vi "PXI_Host_Cluster_Read_NewMethod_Benchmark.vi"() -> ()   [LabVIEW 2018]
uses:
  cRIO RT/TypeDefs/Simple cluster.ctl
  7e8a9f0d-2b7c-4c85-8fb4-747e2fea878c.vi
  cRIO RT/FPGA Bitfile Register Operations/Scalar IO Operations/SubVIs/Convert Cluster BLOB to Bool Array.vi
  cRIO RT/FPGA Bitfile Register Operations/Scalar IO Operations/SubVIs/Parse Cluster Configuration.vi
  cRIO RT/FPGA Bitfile Register Operations/Scalar IO Operations/Read Methods/Read Data Register/Instances/Read U8 Array.vi
  7e8a9f0d-2b7c-4c85-8fb4-747e2fea878c.vi/98fed1db-7537-4d17-af2e-83a63eeec4d6.vi
  cRIO RT/FPGA Bitfile Register Operations/Scalar IO Operations/SubVIs/Check Cluster Configuration Store.vi
  cRIO RT/FPGA Bitfile Register Operations/Scalar IO Operations/Utilities/Find Register Offset.vi
  cRIO RT/FPGA Bitfile Register Operations/Scalar IO Operations/SubVIs/FXP Raw to DBL.vi
  cRIO RT/FPGA Bitfile Register Operations/Scalar IO Operations/SubVIs/Check Register Data Store.vi
  <userlib>/_OpenG.lib/lvdata/lvdata.llb/Variant to Header Info__ogtk.vi
  <userlib>/_OpenG.lib/lvdata/lvdata.llb/Split Cluster TD__ogtk.vi
  <userlib>/_OpenG.lib/lvdata/lvdata.llb/Cluster to Array of VData__ogtk.vi
  <vilib>/Utility/Data Type/Get Type Information.vi
  <userlib>/_OpenG.lib/lvdata/lvdata.llb/Get Strings from Enum__ogtk.vi
  cRIO RT/FPGA Bitfile Register Operations/Scalar IO Operations/Error Handling/Error 6004.vi
  <vilib>/Utility/Data Type/Get Fixed-Point Information.vi
  cRIO RT/FPGA Bitfile Register Operations/Scalar IO Operations/Error Handling/Error 6001.vi
  cRIO RT/FPGA Bitfile Register Operations/Scalar IO Operations/Error Handling/Error 6000.vi
  cRIO RT/FPGA Bitfile Register Operations/Scalar IO Operations/Error Handling/Error 6002.vi
  cRIO RT/FPGA Bitfile Register Operations/Scalar IO Operations/Error Handling/Error 6003.vi
  <vilib>/FPGAPlugInAG/Dynamic/niLvFpga_Close_Dynamic.vi
  <vilib>/rvi/interface/nirviCloseFPGA/nirviCloseFPGA.xnode
  cRIO RT/FPGA Bitfile Register Operations/Scalar IO Operations/FPGA Register IO.lvlib
panel:
  out "error out":errorcluster
  out "Value out":T1
  out "Execution time (s)":dbl
  # "Recorded time"
  # "3.37551E-5"
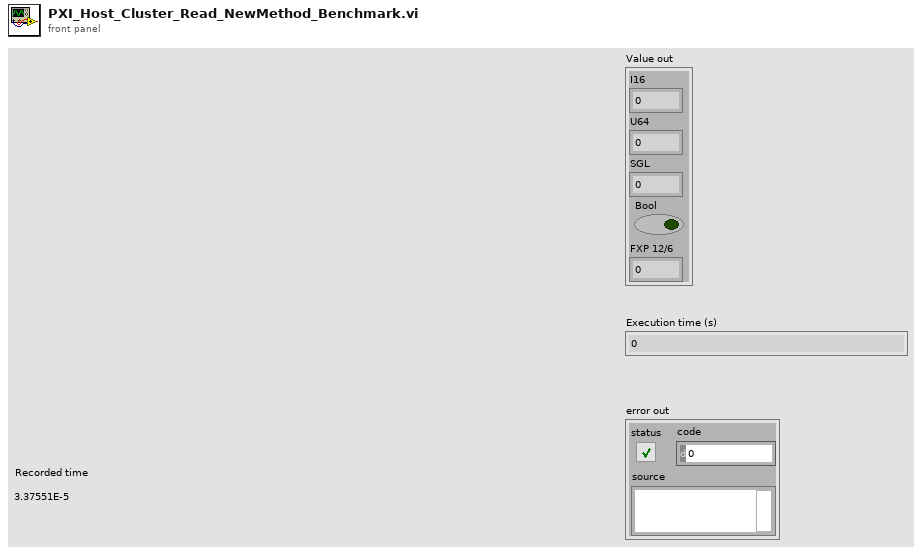
[diagram p1: front panel]
types:
  T1 = typedef "Simple cluster.ctl" = cluster{"I16":i16, "U64":u64, "SGL":sgl, "Bool":bool, "FXP 12/6":fxp<+/-,12,6>}
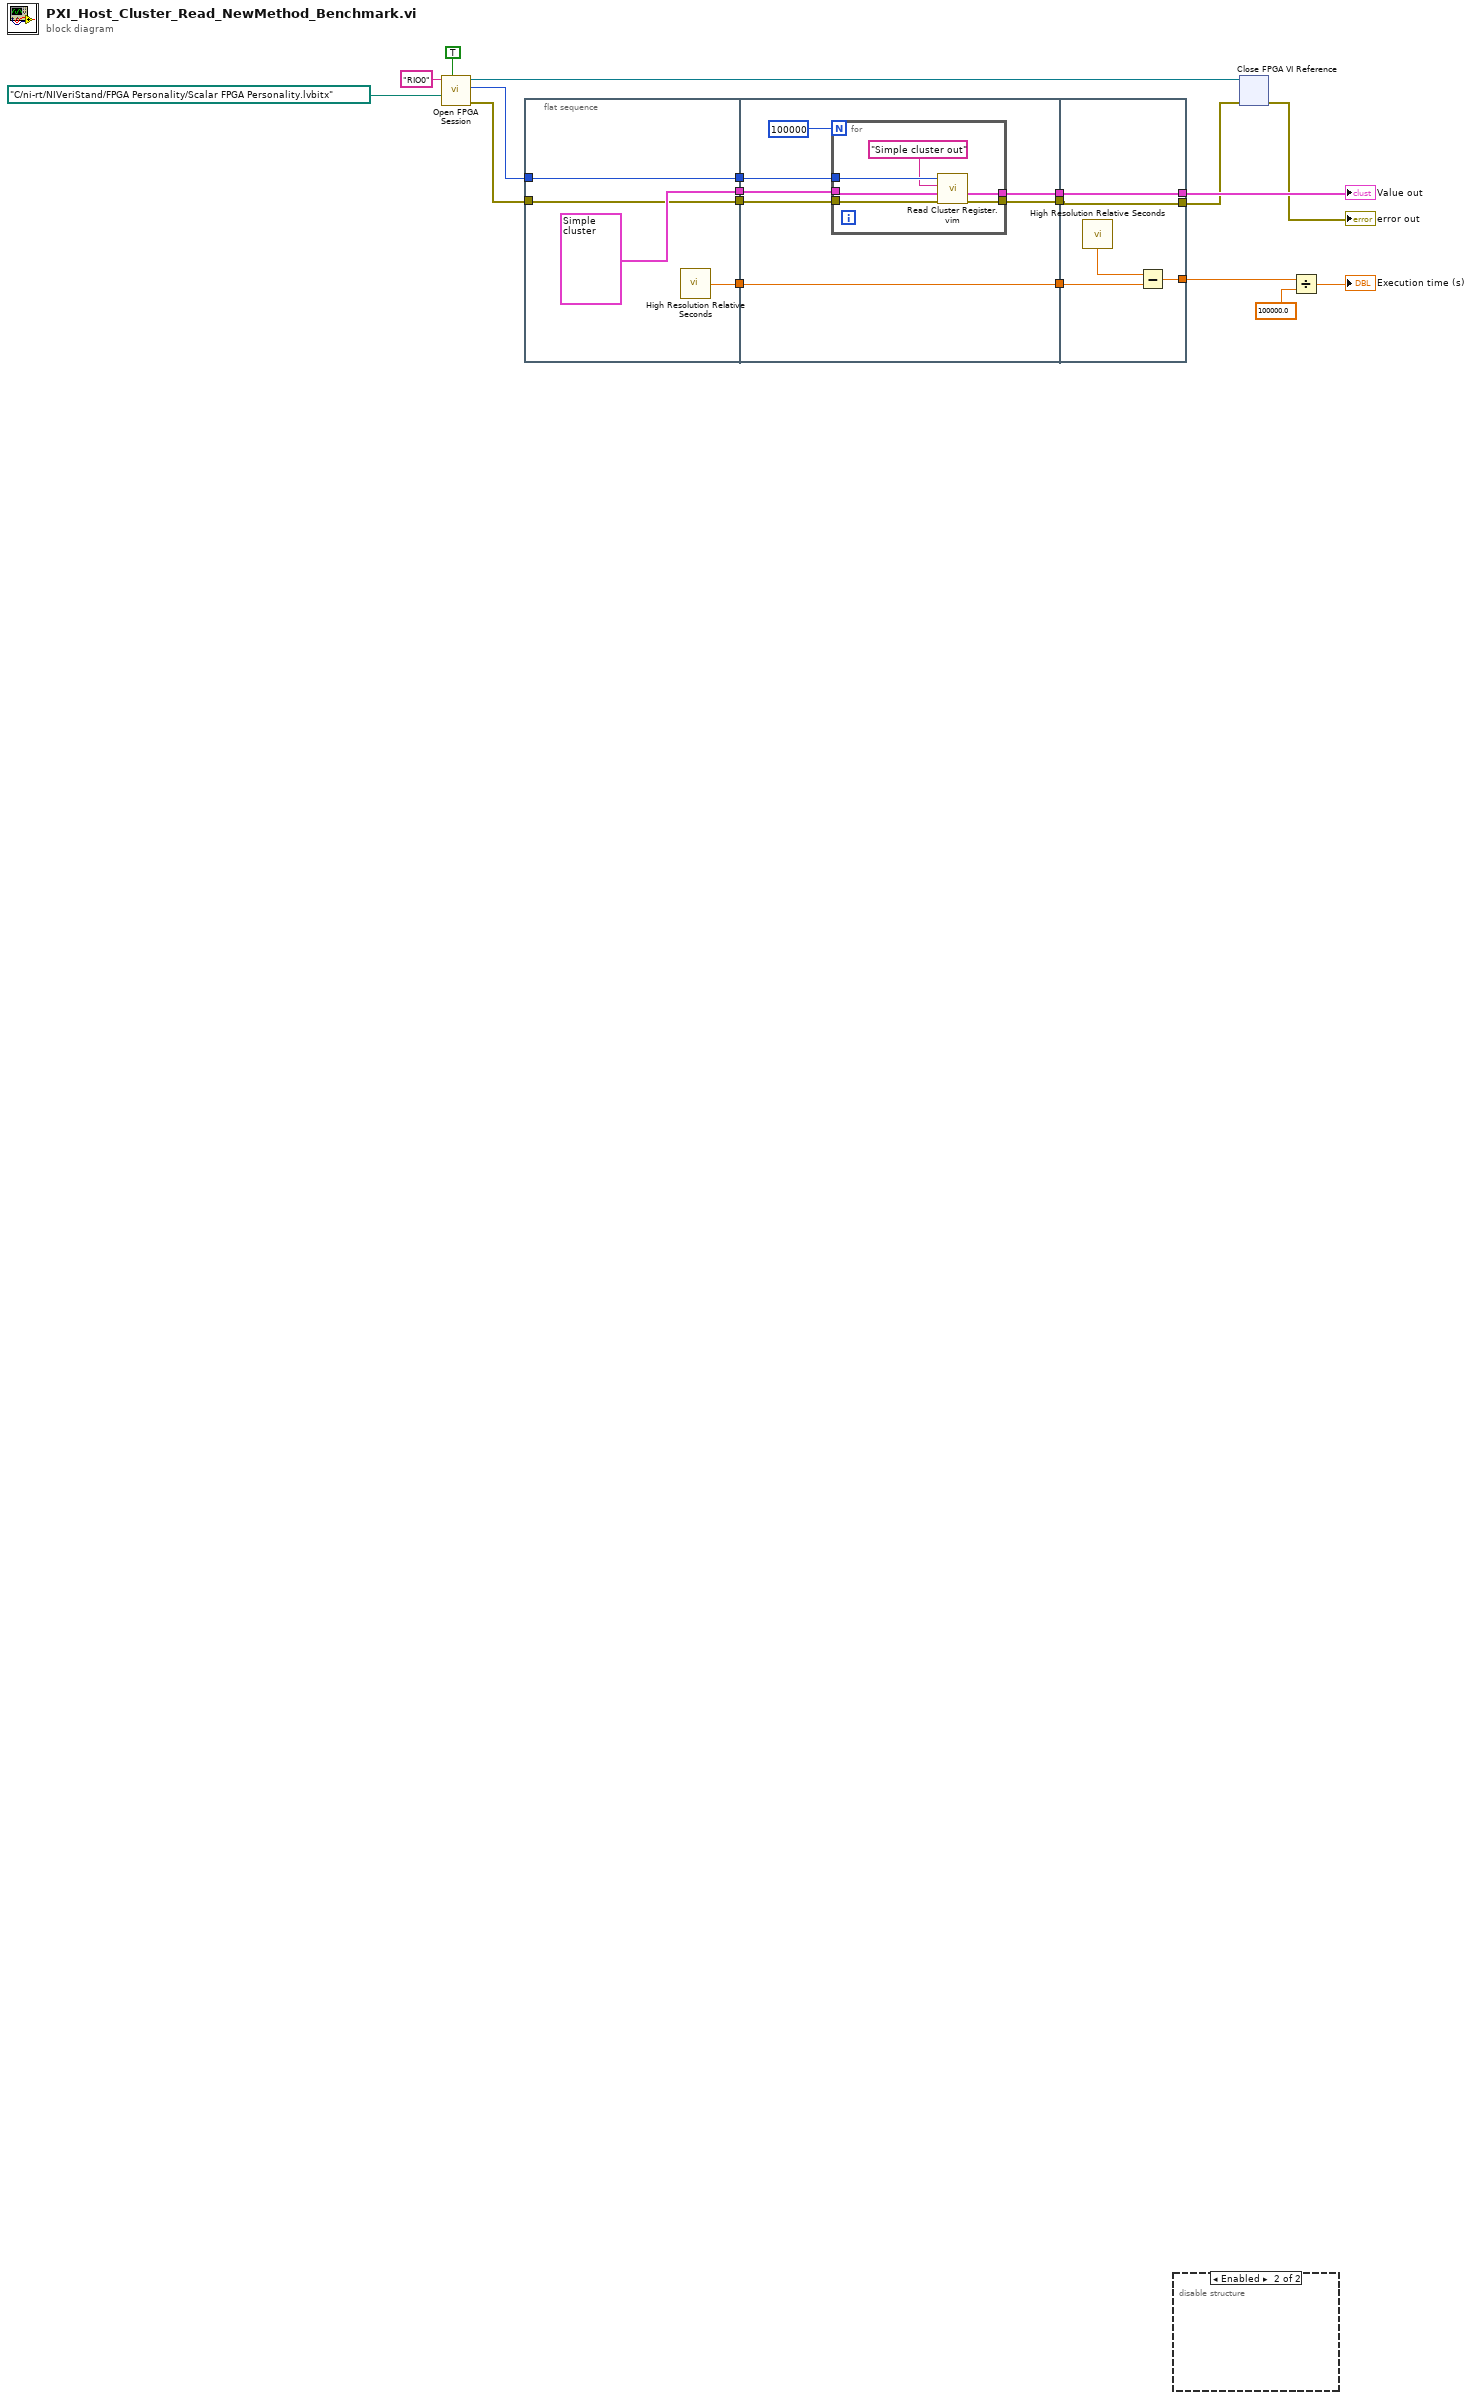
[diagram p0: block diagram]
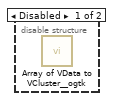
[diagram p2: hidden frame]
diagram:
  n1 = call "Open FPGA Session.vi"("run when loaded (T)"=TRUE, "bitfile path"=path "C:/ni-rt/NIVeriStand/FPGA Personality/Scalar FPGA Personality.lvbitx", "device address"="RIO0") -> ("error out"=w7:errorcluster, "session out"=w12:u32, "bitfile reference out"=w3:refnum<k20>)  [unwired: 6 in]
  n2 = flat-sequence {
    tunnel: [T1 {"I16"=1231, "U64"=213123, "SGL"=1.0, "Bool"=TRUE, "FXP 12/6"=31.984375} ("Simple Cluster")] -> w19
    tunnel: [w22] -> w17
    tunnel: w12 -> [w21]
    tunnel: [w21] -> w11
    tunnel: w7 -> [w20]
    tunnel: [w20] -> w6
    tunnel: w19 -> [w29]
    tunnel: [w28] -> w18
    tunnel: w17 -> [w28]
    tunnel: [w27] -> w13
    tunnel: w11 -> [w26]
    tunnel: w6 -> [w25]
    tunnel: [w24] -> w5
    tunnel: w18 -> [w40]
    tunnel: [w39] -> w16
    tunnel: w13 -> [w38]
    tunnel: w5 -> [w37]
    tunnel: [w38] -> w4
    tunnel: [w37] -> w2
    frame #0 {
      n3 = call <vilib>:"High Resolution Relative Seconds.vi"() -> ("relative seconds"=w22:dbl)
    }
    frame #1 {
      n4 = for {
        N: 100000 -> [_]
        tunnel: w29 -> [w34]
        tunnel: [w31] -> w27
        tunnel: w26 -> [w36]
        tunnel: w25 -> [w33]
        tunnel: [w32] -> w24
        n5 = call "Read Cluster Register.vim"("error in (no error)"=w33, "Cluster in (default value)"=w34, "Cluster Name"="Simple cluster out", "session in"=w36) -> ("error out"=w32:errorcluster, "Cluster out"=w31:T1)  [unwired: 5 in, 1 out]
      }
    }
    frame #2 {
      n6 = call <vilib>:"High Resolution Relative Seconds.vi"() -> ("relative seconds"=w41:dbl)
      n7 = Subtract(x=w41, y=w40) -> (x-y=w39:dbl)
    }
  }
  n8 = disable-structure shown="Enabled" {
    frame Disabled {
      n9 = call <userlib>:"Array of VData to VCluster__ogtk.vi"() -> ()  [unwired: 10 in, 2 out]
    }
    frame Enabled {
    }
  }
  n10 = xnode "Close FPGA VI Reference"("FPGA VI Reference In"=w3, "error in"=w2) -> ("error out"=→"error out":errorcluster)
  n11 = Divide(x=w16, y=100000.0) -> (x/y=→"Execution time (s)":dbl)
  "Value out" <- w4
